vi "ScaleTo16Bit_IQ.vi"(8 "valid in":bool, 10 "factor":u16, 11 "IQ":T1) -> (0 "valid out":bool, 3 "32bit integer":u32)   [LabVIEW 2025]
uses:
  <instrlib>/_niInstr/DSP/v1/Shared/Public/IQ Data.ctl
  <instrlib>/_niInstr/DSP/v1/Shared/niInstr DSP v1 Shared.lvlib
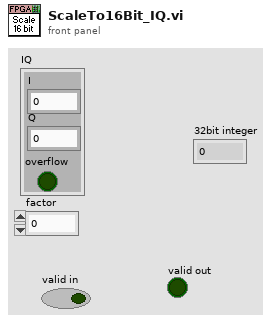
[diagram p1: front panel]
types:
  T1 = typedef "niInstr DSP v1 Shared.lvlib/IQ Data.ctl" = cluster{"I":fxp<+/-,18,1>, "Q":fxp<+/-,18,1>, "overflow":bool}
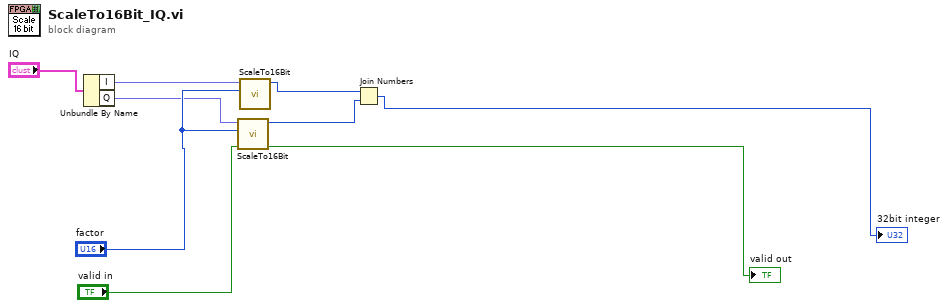
[diagram p0: block diagram]
diagram:
  n1 = Unbundle By Name("IQ") -> ("I"=w8:fxp<+/-,18,1>, "Q"=w6:fxp<+/-,18,1>)
  n2 = call "ScaleTo16Bit.vi"("valid in"="valid in", "factor"="factor", "val"=w6) -> ("valid out"=→"valid out":bool, "16bit integer"=w4:i16)  [unwired: 7 in]
  n3 = call "ScaleTo16Bit.vi"("factor"="factor", "val"=w8) -> ("16bit integer"=w5:i16)  [unwired: 8 in, 1 out]
  n4 = Join Numbers(hi=w5, lo=w4) -> ((hi.lo)=→"32bit integer":u32)
